vi "CreateListImp.vi"(8 "error in (no error)":errorcluster, 11 "List in":refnum<class "List.lvclass">) -> (0 "error out":errorcluster, 3 "List out":refnum<class "List.lvclass">)   [LabVIEW 2017, in "LapDog.Collections.v0.Lists.lvlib" / "List.lvclass"]
uses:
  List.lvclass
  List.lvclass/List.ctl
  ListImp/ListImp.lvclass
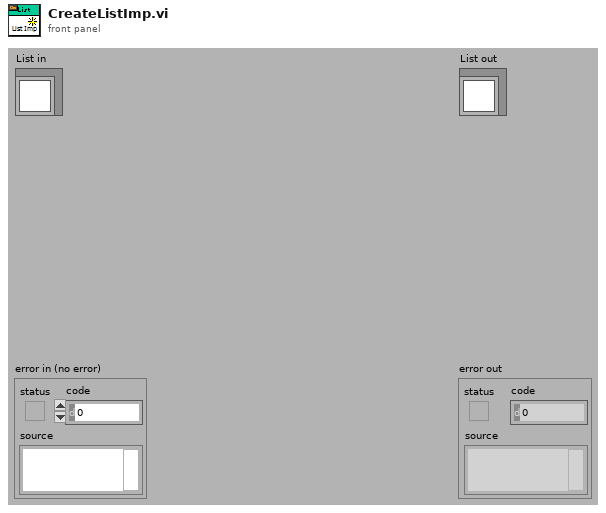
[diagram p1: front panel]
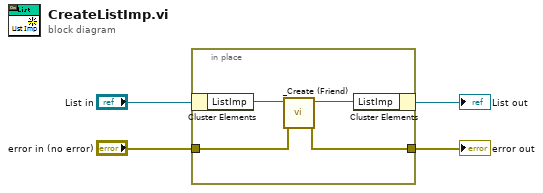
[diagram p0: block diagram]
diagram:
  n1 = in-place {
    in-place-border: "error in (no error)" -> [w6]
    in-place-border: [w5] -> w1
    n2 = in-place-cluster #1("List in") -> ("ListImp"=w8:refnum<class "ListImp.lvclass">)
    n3 = call "_Create (Friend).vi"("error in (no error)"=w6, "ListImp in"=w8) -> ("error out"=w5:errorcluster, "ListImp out"=w7:refnum<class "ListImp.lvclass">)  [unwired: 8 in]
    n4 = in-place-cluster #1("ListImp"=w7) -> (→"List out":refnum<class "List.lvclass">)
  }
  "error out" <- w1
